vi "Release Session.vi"(0 "Session Handle":T1, 11 "error in (no error)":errorcluster, 13 "force destroy? (F)":bool) -> (15 "error out":errorcluster)   [LabVIEW 2014]
doc: "Closes the serial port once all sessions have been released."
uses:
  Typedefs/Session Handle.ctl
  Serial Session.lvclass
  <userlib>/_Session Fwk/Session - Root.lvclass
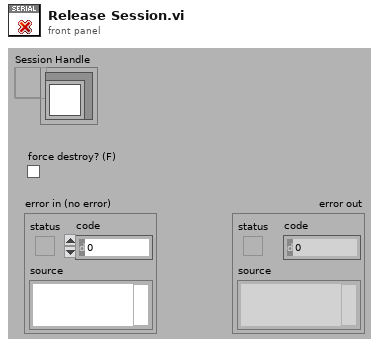
[diagram p1: front panel]
types:
  T1 = typedef "Serial Session.lvclass/Session Handle.ctl" = refnum<data-value>
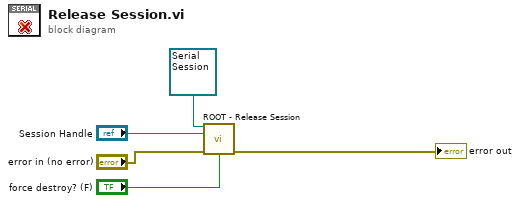
[diagram p0: block diagram]
diagram:
  n1 = call <userlib>:"ROOT - Release Session.vi"("OBJ - Session in"=refnum<class "Serial Session.lvclass"> refnum ("Session class"), "Session Handle in"="Session Handle", "error in (no error)"="error in (no error)", "force destroy? (F)"="force destroy? (F)") -> ("error out"=→"error out":errorcluster)  [unwired: 9 in, 2 out]
